vi "putAirData.vi"(8 "error in (no error)":errorcluster, 10 "TelemetryAirData":T1, 11 "M1M3SAL in":refnum<class "M1M3SAL.lvclass">) -> (0 "error out":errorcluster, 3 "M1M3SAL out":refnum<class "M1M3SAL.lvclass">)   [LabVIEW 2016, in "M1M3SupportCommunicator.lvlib" / "M1M3SAL.lvclass"]
uses:
  M1M3SAL.lvclass
  DataTypes/Topics/TelemetryAirData.ctl
  DataTypes/Topics/Parts/Timestamp.ctl
  DataTypes/MessageHeader.ctl
  DataTypes/MessageTypes.ctl
  DataTypes/MessageTopics.ctl
  Common_RT_Utilities/U8ArrayBuilderAutoIndexing/U8ArrayBuilderAutoIndexing.lvclass
  M1M3SupportCommunicator.lvlib
  DataTypes/Topics/M1M3SupportTopics.lvlib
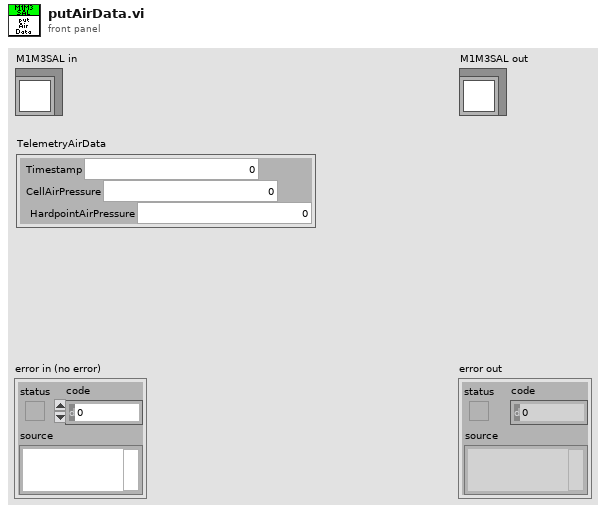
[diagram p1: front panel]
types:
  T1 = typedef "M1M3SupportTopics.lvlib/TelemetryAirData.ctl" = cluster{"Timestamp":T2, "CellAirPressure":sgl, "HardpointAirPressure":sgl}
  T2 = typedef "M1M3SupportTopics.lvlib/Timestamp.ctl" = dbl
  T3 = typedef "M1M3SupportCommunicator.lvlib/MessageHeader.ctl" = cluster{"Type":T4, "Topic":T5, "Size":i32}
  T4 = typedef "M1M3SupportCommunicator.lvlib/MessageTypes.ctl" = enum8{"None", "PutSample", "GetNextSample", "LogEvent", "GetEvent", "IssueCommand", "CommandId", "WaitForCompletion", "AcceptCommand", "AckCommand"}
  T5 = typedef "M1M3SupportCommunicator.lvlib/MessageTopics.ctl" = enum8{"None", "ForceActuatorData", "MirrorForceData", "HardpointData", "AirData", "DynamicData", "FPGAData", "IMSData", "ForceActuatorStatus", "ElevationData", "HardpointStatus", "HardpointActuatorChase", "AirStatus", "ForceActuatorSafetyChecks", "ForceActuatorTest", "ActuatorBroadcastCounter", "StatusChecks", "CellChecks", "HardpointActuatorBreakaway", "RaiseMirrorComplete", "ILCCommunication", "ElevationAngleChecks", "DetailedState", "ServoLoops", "ForceActuatorInfo", "LowerMirrorComplete", "HardpointActuatorInfo", "SettingsApplied", "ErrorCode", "StartupChecks", "SummaryState", "SettingVersions", "ActuatorTestStatus", "AppliedSettingsMatchStart", "Enable", "EnterMaintenance", "Standby", "AbortLowerM1M3", "ApplyAberrationByForces", "ApplyAOSCorrectionByBendingModes", "ClearAOSCorrection", "Start", "RaiseM1M3", "TestForceActuator", "LowerM1M3", "ApplyAOSCorrectionByForces", "Disable", "ApplyAberationByBendingMode", "TestHardpoint", "ManipulateM1M3", "ClearAberration", "Exit", "TestAir", "AbortRaiseM1M3", "MoveHardpointActuators", "ExitMaintenance", "Shutdown"}
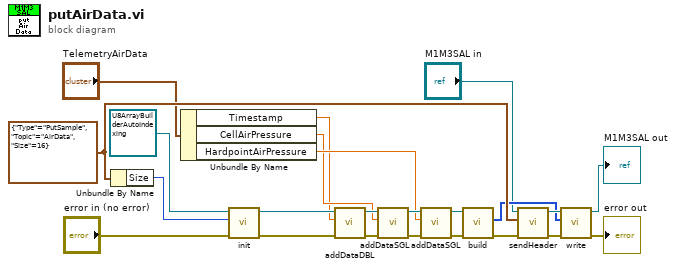
[diagram p0: block diagram]
diagram:
  w22 = T3 {"Type"=enum."PutSample", "Topic"=enum."AirData", "Size"=16} ("MessageHeader")
  n1 = Unbundle By Name(w22) -> ("Size"=w21:i32)
  n2 = Unbundle By Name("TelemetryAirData") -> ("Timestamp"=w1:T2, "CellAirPressure"=w2:sgl, "HardpointAirPressure"=w3:sgl)
  n3 = call "init.vi"("error in (no error)"="error in (no error)", "Size"=w21, "U8ArrayBuilderAutoIndexing in"=refnum<class "U8ArrayBuilderAutoIndexing.lvclass"> refnum ("RTUtilities.lvlib:U8ArrayBuilderAutoIndexing.lvclass")) -> ("error out"=w11:errorcluster, "U8ArrayBuilderAutoIndexing out"=w12:refnum<class "U8ArrayBuilderAutoIndexing.lvclass">)  [unwired: 7 in]
  n4 = call "addDataDBL.vi"("error in (no error)"=w11, "Data"=w1, "U8ArrayBuilderAutoIndexing in"=w12) -> ("error out"=w6:errorcluster, "U8ArrayBuilderAutoIndexing out"=w7:refnum<class "U8ArrayBuilderAutoIndexing.lvclass">)  [unwired: 7 in]
  n5 = call "addDataSGL.vi"("error in (no error)"=w6, "Data"=w2, "U8ArrayBuilderAutoIndexing in"=w7) -> ("error out"=w9:errorcluster, "U8ArrayBuilderAutoIndexing out"=w8:refnum<class "U8ArrayBuilderAutoIndexing.lvclass">)  [unwired: 7 in]
  n6 = call "addDataSGL.vi"("error in (no error)"=w9, "Data"=w3, "U8ArrayBuilderAutoIndexing in"=w8) -> ("error out"=w4:errorcluster, "U8ArrayBuilderAutoIndexing out"=w5:refnum<class "U8ArrayBuilderAutoIndexing.lvclass">)  [unwired: 7 in]
  n7 = call "build.vi"("error in (no error)"=w4, "U8ArrayBuilderAutoIndexing in"=w5) -> ("error out"=w18:errorcluster, "Array"=w19:u8[])  [unwired: 7 in, 1 out]
  n8 = call "sendHeader.vi"("error in (no error)"=w18, "MessageHeader"=w22, "M1M3SAL in"="M1M3SAL in") -> ("error out"=w17:errorcluster, "M1M3SAL out"=w20:refnum<class "M1M3SAL.lvclass">)  [unwired: 7 in]
  n9 = call "write.vi"("error in (no error)"=w17, "Data"=w19, "M1M3SAL in"=w20) -> ("error out"=→"error out":errorcluster, "M1M3SAL out"=→"M1M3SAL out":refnum<class "M1M3SAL.lvclass">)  [unwired: 7 in]
